vi "Read AI and Write AO.vi"(8 "error in (no error)":errorcluster, 10 "AO []":waveform(dbl)[](array[waveform]), 11 "LockinDAQ":refnum<class "LockinDAQ.lvclass">) -> (0 "error out":errorcluster, 2 "AI []":waveform(dbl)[](array[waveform]), 3 "LockinDAQ out":refnum<class "LockinDAQ.lvclass">)   [LabVIEW 2016, in "LockinDAQ.lvclass"]
uses:
  LockinDAQ.lvclass
  LockinDAQ.lvclass/LockinDAQ.ctl
  Typedefs/DAQType-enum.ctl
  <vilib>/DAQmx/write.llb/DAQmx Write (Analog 1D Wfm NChan NSamp).vi
  <vilib>/DAQmx/read.llb/DAQmx Read (Analog 1D Wfm NChan NSamp).vi
  <vilib>/DAQmx/miscellaneous.llb/DAQmx Fill In Error Info.vi
  <resource>/objmgr/daqmx.rc
panel:
  out "Numeric":i32
  out "AvailSampPerChan 4":u32
  out "AvailSampPerChan 3":u32
  out "AvailSampPerChan 2":u32
  out "AvailSampPerChan 1":u32
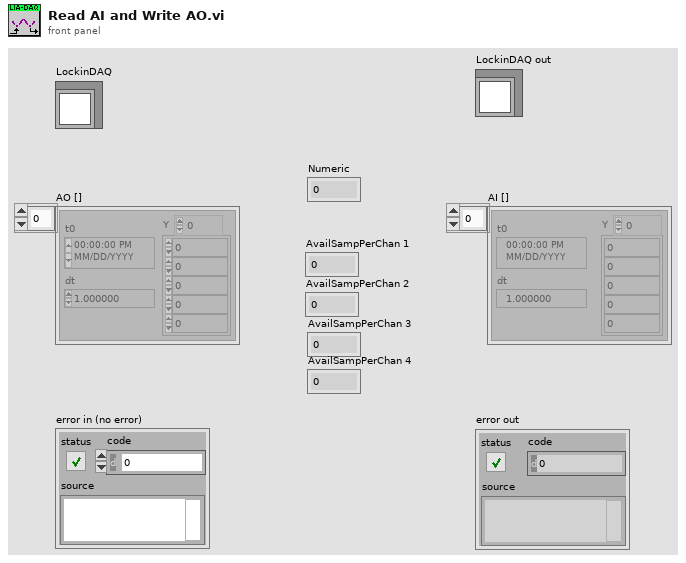
[diagram p1: front panel]
types:
  T1 = typedef "LockinDAQ.lvclass/DAQType-enum.ctl" = enum16{"None", "USB 4431", "PXI 446x"}
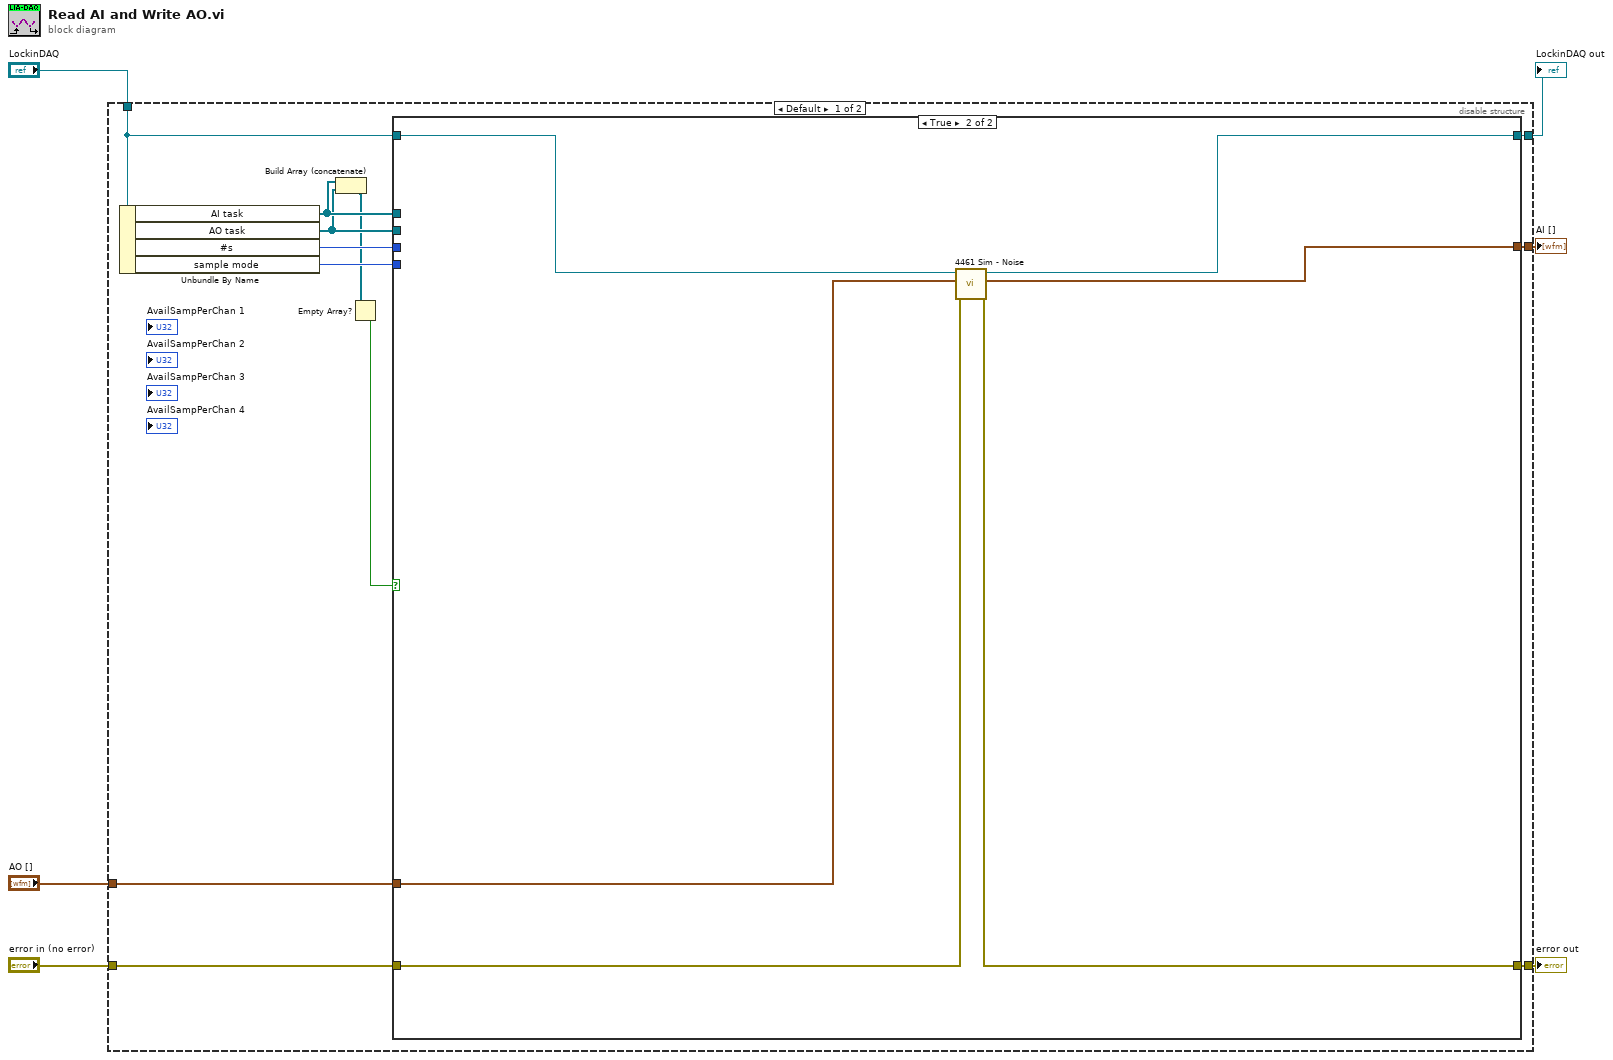
[diagram p0: block diagram]
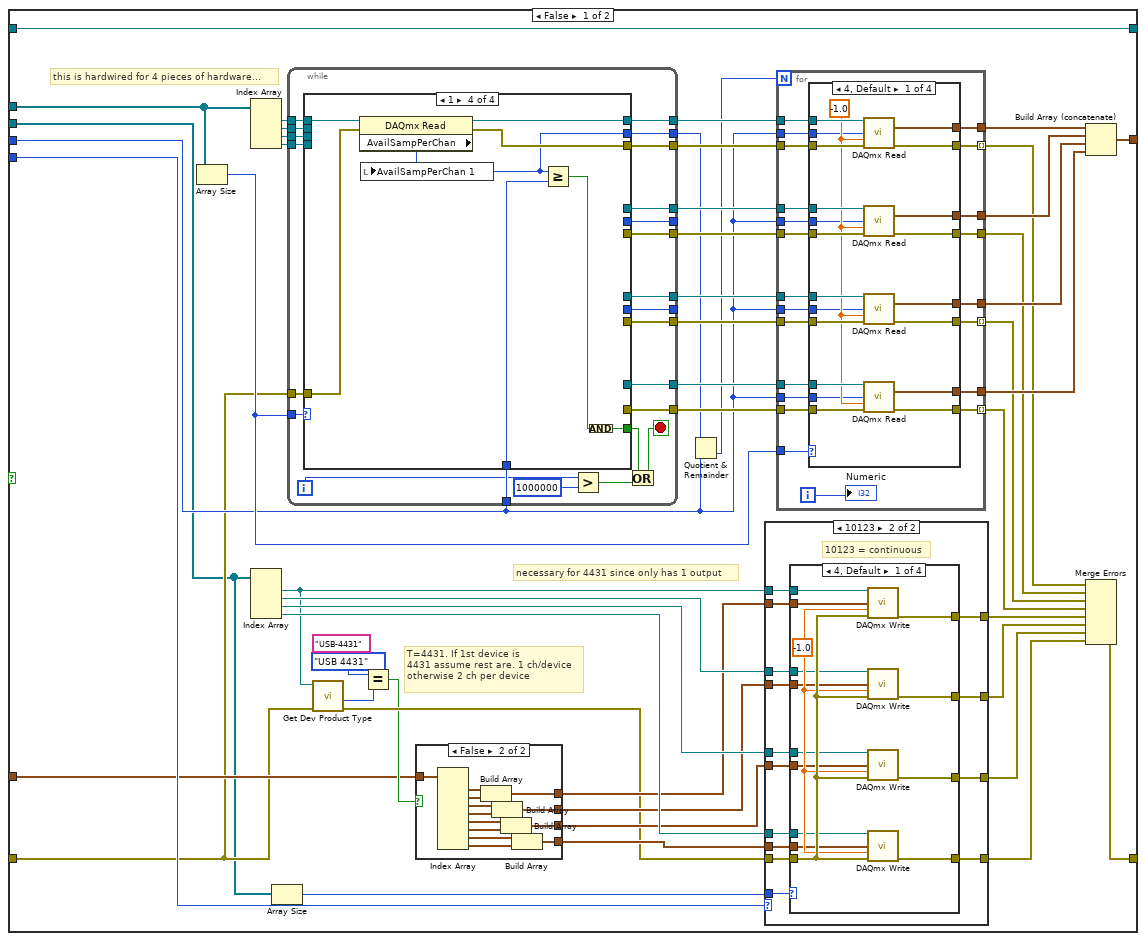
[diagram p2: hidden frame]
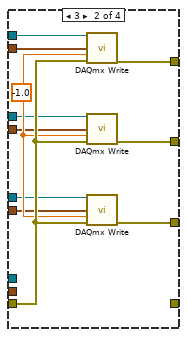
[diagram p4: hidden frame]
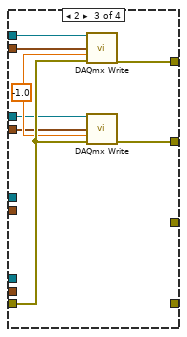
[diagram p5: hidden frame]
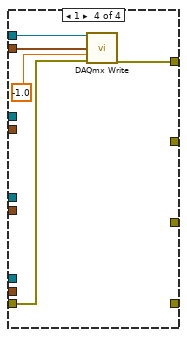
[diagram p6: hidden frame]
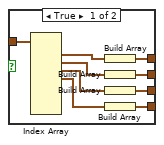
[diagram p7: hidden frame]
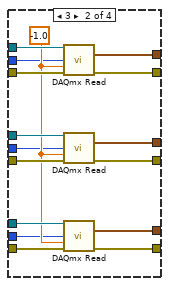
[diagram p8: hidden frame]
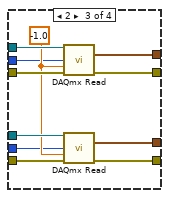
[diagram p9: hidden frame]
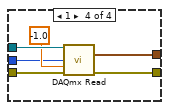
[diagram p10: hidden frame]
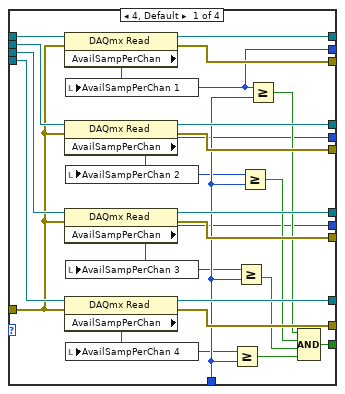
[diagram p11: hidden frame]
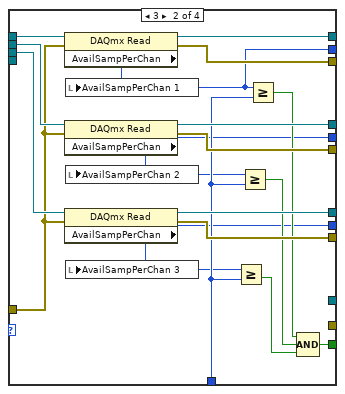
[diagram p12: hidden frame]
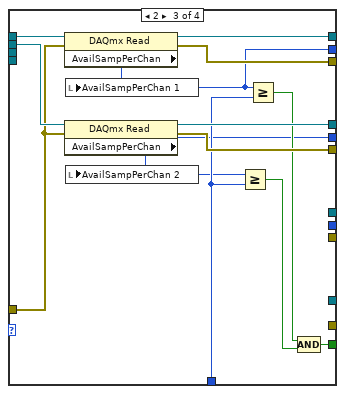
[diagram p13: hidden frame]
diagram:
  n1 = disable-structure shown="Default" {
    disable-tunnel: [w18 w309] -> w6
    disable-tunnel: [w15 w310] -> w5
    disable-tunnel: "LockinDAQ" -> [w8 _]
    disable-tunnel: "AO []" -> [w14 w309]
    disable-tunnel: "error in (no error)" -> [w13 w310]
    disable-tunnel: [w7 _] -> w1
    frame condition #0 (active) {
      n2 = Unbundle By Name(w8) -> ("AI task"=w12:refnum<k21>[], "AO task"=w11:refnum<k21>[], "#s"=w17:i32, "sample mode"=w16:i32)
      n3 = Build Array (concatenate)(w12, w11) -> (w10:refnum<k21>[])
      n4 = Empty Array?(array=w10) -> (empty?=w9:bool)
      n5 = case shown="True" w9 {
        tunnel: [w67 w306] -> w18
        tunnel: w17 -> [w29 _]
        tunnel: w16 -> [w28 _]
        tunnel: [w27 w304] -> w15
        tunnel: w14 -> [w26 w303]
        tunnel: w13 -> [w25 w305]
        tunnel: w12 -> [w21 _]
        tunnel: w11 -> [w20 _]
        tunnel: w8 -> [w19 w308]
        tunnel: [w19 w307] -> w7
        frame False {
          (unwired) "USB-4431" ("ProductType")
          # "this is hardwired for 4 pieces of hardware..."
          # "T=4431. If 1st device is \n4431 assume rest are. 1 ch/device\notherwise 2 ch per device"
          # "necessary for 4431 since only has 1 output"
          n6 = Array Size(array=w21) -> (size(s)=w35:i32)
          n7 = Index Array(array=w21) -> (element #1=w63:refnum<k21>, element #2=w64:refnum<k21>, element #3=w65:refnum<k21>, element #4=w66:refnum<k21>)  [unwired: 4 in]
          n8 = Index Array(array=w20) -> (element #1=w43:refnum<k21>, element #2=w54:refnum<k21>, element #3=w53:refnum<k21>, element #4=w52:refnum<k21>)  [unwired: 4 in]
          n9 = Array Size(array=w20) -> (size(s)=w44:i32)
          n10 = while {
            tunnel: w66 -> [w240]
            tunnel: w65 -> [w239]
            tunnel: w64 -> [w238]
            tunnel: w63 -> [w237]
            tunnel: [w236] -> w62
            tunnel: [w235] -> w61
            tunnel: [w234] -> w60
            tunnel: [w233] -> w59
            tunnel: w25 -> [w228]
            tunnel: [w232] -> w58
            tunnel: [w231] -> w57
            tunnel: [w230] -> w56
            tunnel: [w229] -> w55
            tunnel: w29 -> [w227]
            tunnel: [w224] -> w45
            tunnel: [w226] -> _
            tunnel: [w225] -> _
            tunnel: w35 -> [w223]
            i -> [w220]
            stop <- w221 stop-if-true
            n11 = case shown="1" w223 {
              tunnel: w240 -> [w263 _ _ _]
              tunnel: w239 -> [w262 w281 _ _]
              tunnel: w238 -> [w261 w280 w294 _]
              tunnel: w237 -> [w260 w279 w293 w302]
              tunnel: [w259 w278 w292 w301] -> w236
              tunnel: [w258 w277 w291 _] -> w235
              tunnel: [w257 w276 _ _] -> w234
              tunnel: [w256 _ _ _] -> w233
              tunnel: [w255 w275 w290 w300] -> w232
              tunnel: [w254 w274 w289 _] -> w231
              tunnel: [w253 w273 _ _] -> w230
              tunnel: [w252 _ _ _] -> w229
              tunnel: w228 -> [w251 w272 w288 w299]
              tunnel: w227 -> [w246 w268 w285 w297]
              tunnel: [w241 w264 w282 w295] -> w222
              tunnel: [w244 w267 _ _] -> w226
              tunnel: [w243 w266 w284 _] -> w225
              tunnel: [w242 w265 w283 w296] -> w224
              frame 4, Default {
                n12 = property class="DAQmx Read"(reference=w260, error in=w251) -> (reference out=w259:refnum<k21>, error out=w255:errorcluster, "AvailSampPerChan"=w242:u32)
                n13 = property class="DAQmx Read"(reference=w261, error in=w251) -> (reference out=w258:refnum<k21>, error out=w254:errorcluster, "AvailSampPerChan"=w243:u32)
                n14 = property class="DAQmx Read"(reference=w262, error in=w251) -> (reference out=w257:refnum<k21>, error out=w253:errorcluster, "AvailSampPerChan"=w244:u32)
                n15 = property class="DAQmx Read"(reference=w263, error in=w251) -> (reference out=w256:refnum<k21>, error out=w252:errorcluster, "AvailSampPerChan"=w245:u32)
                n16 = local write "AvailSampPerChan 1"(w242) -> ()
                n17 = local write "AvailSampPerChan 2"(w243) -> ()
                n18 = local write "AvailSampPerChan 3"(w244) -> ()
                n19 = local write "AvailSampPerChan 4"(w245) -> ()
                n20 = Greater Or Equal?(x=w245, y=w246) -> (x >= y?=w250:bool)
                n21 = Greater Or Equal?(x=w244, y=w246) -> (x >= y?=w249:bool)
                n22 = Greater Or Equal?(x=w243, y=w246) -> (x >= y?=w248:bool)
                n23 = Greater Or Equal?(x=w242, y=w246) -> (x >= y?=w247:bool)
                n24 = Compound Arithmetic op=AND(w247, w248, w249, w250) -> (w241:bool)
              }
              frame 3 {
                n25 = property class="DAQmx Read"(reference=w279, error in=w272) -> (reference out=w278:refnum<k21>, error out=w275:errorcluster, "AvailSampPerChan"=w265:u32)
                n26 = property class="DAQmx Read"(reference=w280, error in=w272) -> (reference out=w277:refnum<k21>, error out=w274:errorcluster, "AvailSampPerChan"=w266:u32)
                n27 = property class="DAQmx Read"(reference=w281, error in=w272) -> (reference out=w276:refnum<k21>, error out=w273:errorcluster, "AvailSampPerChan"=w267:u32)
                n28 = local write "AvailSampPerChan 1"(w265) -> ()
                n29 = local write "AvailSampPerChan 2"(w266) -> ()
                n30 = local write "AvailSampPerChan 3"(w267) -> ()
                n31 = Greater Or Equal?(x=w267, y=w268) -> (x >= y?=w271:bool)
                n32 = Greater Or Equal?(x=w266, y=w268) -> (x >= y?=w270:bool)
                n33 = Greater Or Equal?(x=w265, y=w268) -> (x >= y?=w269:bool)
                n34 = Compound Arithmetic op=AND(w269, w270, w271) -> (w264:bool)
              }
              frame 2 {
                n35 = property class="DAQmx Read"(reference=w293, error in=w288) -> (reference out=w292:refnum<k21>, error out=w290:errorcluster, "AvailSampPerChan"=w283:u32)
                n36 = property class="DAQmx Read"(reference=w294, error in=w288) -> (reference out=w291:refnum<k21>, error out=w289:errorcluster, "AvailSampPerChan"=w284:u32)
                n37 = local write "AvailSampPerChan 1"(w283) -> ()
                n38 = local write "AvailSampPerChan 2"(w284) -> ()
                n39 = Greater Or Equal?(x=w284, y=w285) -> (x >= y?=w287:bool)
                n40 = Greater Or Equal?(x=w283, y=w285) -> (x >= y?=w286:bool)
                n41 = Compound Arithmetic op=AND(w286, w287) -> (w282:bool)
              }
              frame 1 {
                n42 = property class="DAQmx Read"(reference=w302, error in=w299) -> (reference out=w301:refnum<k21>, error out=w300:errorcluster, "AvailSampPerChan"=w296:u32)
                n43 = local write "AvailSampPerChan 1"(w296) -> ()
                n44 = Greater Or Equal?(x=w296, y=w297) -> (x >= y?=w298:bool)
                n45 = Compound Arithmetic op=AND(w298) -> (w295:bool)
              }
            }
            n46 = Greater?(x=w220, y=1000000) -> (0:w218:bool)
            n47 = Or(x=w222, y=w218) -> (x .or. y?=w221:bool)
          }
          n48 = call "Get Dev Product Type.vi"("error in (no error)"=w25, "Refnum in"=w43) -> ("error out"=w37:errorcluster, "DAQ Type"=w38:T1)  [unwired: 6 in, 2 out]
          n49 = Equal?(x=DAQType-enum."USB 4431", y=w38) -> (x = y?=w36:bool)
          n50 = case shown="False" w36 {
            tunnel: [w128 w134] -> w40
            tunnel: [w127 w133] -> w41
            tunnel: [w126 w132] -> w42
            tunnel: [w124 w130] -> w39
            tunnel: w26 -> [w123 w129]
            frame True {
              n51 = Index Array(array=w123) -> (element #1=w125:waveform(dbl), element #2=w122:waveform(dbl), element #3=w121:waveform(dbl), element #4=w120:waveform(dbl))  [unwired: 8 in, 4 out]
              n52 = Build Array(w125) -> (w124:waveform(dbl)[])
              n53 = Build Array(w122) -> (w128:waveform(dbl)[])
              n54 = Build Array(w121) -> (w127:waveform(dbl)[])
              n55 = Build Array(w120) -> (w126:waveform(dbl)[])
            }
            frame False {
              n56 = Index Array(array=w129) -> (element #1=w131:waveform(dbl), element #2=w141:waveform(dbl), element #3=w140:waveform(dbl), element #4=w139:waveform(dbl), element #5=w138:waveform(dbl), element #6=w137:waveform(dbl), element #7=w136:waveform(dbl), element #8=w135:waveform(dbl))  [unwired: 8 in]
              n57 = Build Array(w131, w141) -> (w130:waveform(dbl)[])
              n58 = Build Array(w140, w139) -> (w134:waveform(dbl)[])
              n59 = Build Array(w138, w137) -> (w133:waveform(dbl)[])
              n60 = Build Array(w136, w135) -> (w132:waveform(dbl)[])
            }
          }
          n61 = Quotient & Remainder(x=w45, y=w29) -> (floor(x/y)=w46:u32)  [unwired: 1 out]
          n62 = case shown="10123" w28 {
            tunnel: w54 -> [_ w81]
            tunnel: w53 -> [_ w80]
            tunnel: w52 -> [_ w79]
            tunnel: [_ w78] -> w51
            tunnel: [_ w77] -> w24
            tunnel: [_ w76] -> w23
            tunnel: [_ w75] -> w22
            tunnel: w44 -> [_ w74]
            tunnel: w43 -> [_ w73]
            tunnel: w42 -> [_ w72]
            tunnel: w41 -> [_ w71]
            tunnel: w40 -> [_ w70]
            tunnel: w39 -> [_ w69]
            tunnel: w37 -> [_ w68]
            frame 10178, Default {
              # "10178 = finite sample mode (IV\nmode). Do not try to write\nmore samples to the buffer"
            }
            frame 10123 {
              # "10123 = continuous"
              n63 = case shown="4, Default" w74 {
                tunnel: w68 -> [w95 w106 w114 w119]
                tunnel: w81 -> [w93 w104 w112 _]
                tunnel: w80 -> [w92 w103 _ _]
                tunnel: w79 -> [w91 _ _ _]
                tunnel: w70 -> [w90 w102 w111 _]
                tunnel: w71 -> [w89 w101 _ _]
                tunnel: w72 -> [w88 _ _ _]
                tunnel: [w87 w100 w110 w117] -> w78
                tunnel: [w86 w99 w109 _] -> w77
                tunnel: [w85 w98 _ _] -> w76
                tunnel: [w84 _ _ _] -> w75
                tunnel: w73 -> [w83 w97 w108 w116]
                tunnel: w69 -> [w82 w96 w107 w115]
                frame 4, Default {
                  w94 = -1.0 ("timeout")
                  n64 = call-poly <vilib>:"DAQmx Write.vi"("task/channels in"=w83, "data"=w82, "timeout"=w94, "error in"=w95) -> ("error out"=w87:errorcluster)  [unwired: 9 in, 2 out]
                  n65 = call-poly <vilib>:"DAQmx Write.vi"("task/channels in"=w93, "data"=w90, "timeout"=w94, "error in"=w95) -> ("error out"=w86:errorcluster)  [unwired: 9 in, 2 out]
                  n66 = call-poly <vilib>:"DAQmx Write.vi"("task/channels in"=w92, "data"=w89, "timeout"=w94, "error in"=w95) -> ("error out"=w85:errorcluster)  [unwired: 9 in, 2 out]
                  n67 = call-poly <vilib>:"DAQmx Write.vi"("task/channels in"=w91, "data"=w88, "timeout"=w94, "error in"=w95) -> ("error out"=w84:errorcluster)  [unwired: 9 in, 2 out]
                }
                frame 3 {
                  w105 = -1.0 ("timeout")
                  n68 = call-poly <vilib>:"DAQmx Write.vi"("task/channels in"=w97, "data"=w96, "timeout"=w105, "error in"=w106) -> ("error out"=w100:errorcluster)  [unwired: 9 in, 2 out]
                  n69 = call-poly <vilib>:"DAQmx Write.vi"("task/channels in"=w104, "data"=w102, "timeout"=w105, "error in"=w106) -> ("error out"=w99:errorcluster)  [unwired: 9 in, 2 out]
                  n70 = call-poly <vilib>:"DAQmx Write.vi"("task/channels in"=w103, "data"=w101, "timeout"=w105, "error in"=w106) -> ("error out"=w98:errorcluster)  [unwired: 9 in, 2 out]
                }
                frame 2 {
                  w113 = -1.0 ("timeout")
                  n71 = call-poly <vilib>:"DAQmx Write.vi"("task/channels in"=w108, "data"=w107, "timeout"=w113, "error in"=w114) -> ("error out"=w110:errorcluster)  [unwired: 9 in, 2 out]
                  n72 = call-poly <vilib>:"DAQmx Write.vi"("task/channels in"=w112, "data"=w111, "timeout"=w113, "error in"=w114) -> ("error out"=w109:errorcluster)  [unwired: 9 in, 2 out]
                }
                frame 1 {
                  n73 = call-poly <vilib>:"DAQmx Write.vi"("task/channels in"=w116, "data"=w115, "timeout"=-1.0, "error in"=w119) -> ("error out"=w117:errorcluster)  [unwired: 9 in, 2 out]
                }
              }
            }
          }
          n74 = for {
            N: w46 -> [_]
            tunnel: w62 -> [w163]
            tunnel: w61 -> [w162]
            tunnel: w60 -> [w161]
            tunnel: w59 -> [w160]
            tunnel: w58 -> [w159]
            tunnel: w57 -> [w158]
            tunnel: w56 -> [w157]
            tunnel: w55 -> [w156]
            tunnel: [w155] -> w50
            tunnel: [w154] -> w49
            tunnel: [w153] -> w48
            tunnel: [w152] -> w47
            tunnel: w29 -> [w151]
            tunnel: w29 -> [w150]
            tunnel: w29 -> [w149]
            tunnel: w29 -> [w148]
            tunnel: [w147] -> w32 mode=indexing
            tunnel: [w146] -> w33
            tunnel: [w145] -> w34 mode=indexing
            tunnel: [w144] -> w31 mode=indexing
            tunnel: w35 -> [w142]
            i -> [w143]
            n75 = case shown="4, Default" w142 {
              tunnel: w163 -> [w184 w200 w211 w217]
              tunnel: w162 -> [w183 w199 w210 _]
              tunnel: w161 -> [w182 w198 _ _]
              tunnel: w160 -> [w181 _ _ _]
              tunnel: w159 -> [w180 w197 w209 w216]
              tunnel: w158 -> [w179 w196 w208 _]
              tunnel: w157 -> [w178 w195 _ _]
              tunnel: w156 -> [w177 _ _ _]
              tunnel: [w175 w193 w206 _] -> w155
              tunnel: [w174 w192 w205 w214] -> w154
              tunnel: [w173 w191 _ _] -> w153
              tunnel: [w172 _ _ _] -> w152
              tunnel: w151 -> [w171 _ _ _]
              tunnel: w150 -> [w170 w190 w204 w213]
              tunnel: w149 -> [w169 w189 _ _]
              tunnel: w148 -> [w168 w188 w203 _]
              tunnel: [w167 w187 w202 w212] -> w147
              tunnel: [w166 w186 w201 _] -> w146
              tunnel: [w165 w185 _ _] -> w145
              tunnel: [w164 _ _ _] -> w144
              frame 4, Default {
                w176 = -1.0 ("timeout")
                n76 = call-poly <vilib>:"DAQmx Read.vi"("task/channels in"=w184, "number of samples per channel"=w170, "timeout"=w176, "error in"=w180) -> ("data"=w174:waveform(dbl)[], "error out"=w167:errorcluster)  [unwired: 9 in, 1 out]
                n77 = call-poly <vilib>:"DAQmx Read.vi"("task/channels in"=w183, "number of samples per channel"=w168, "timeout"=w176, "error in"=w179) -> ("data"=w175:waveform(dbl)[], "error out"=w166:errorcluster)  [unwired: 9 in, 1 out]
                n78 = call-poly <vilib>:"DAQmx Read.vi"("task/channels in"=w182, "number of samples per channel"=w169, "timeout"=w176, "error in"=w178) -> ("data"=w173:waveform(dbl)[], "error out"=w165:errorcluster)  [unwired: 9 in, 1 out]
                n79 = call-poly <vilib>:"DAQmx Read.vi"("task/channels in"=w181, "number of samples per channel"=w171, "timeout"=w176, "error in"=w177) -> ("data"=w172:waveform(dbl)[], "error out"=w164:errorcluster)  [unwired: 9 in, 1 out]
              }
              frame 3 {
                w194 = -1.0 ("timeout")
                n80 = call-poly <vilib>:"DAQmx Read.vi"("task/channels in"=w200, "number of samples per channel"=w190, "timeout"=w194, "error in"=w197) -> ("data"=w192:waveform(dbl)[], "error out"=w187:errorcluster)  [unwired: 9 in, 1 out]
                n81 = call-poly <vilib>:"DAQmx Read.vi"("task/channels in"=w199, "number of samples per channel"=w188, "timeout"=w194, "error in"=w196) -> ("data"=w193:waveform(dbl)[], "error out"=w186:errorcluster)  [unwired: 9 in, 1 out]
                n82 = call-poly <vilib>:"DAQmx Read.vi"("task/channels in"=w198, "number of samples per channel"=w189, "timeout"=w194, "error in"=w195) -> ("data"=w191:waveform(dbl)[], "error out"=w185:errorcluster)  [unwired: 9 in, 1 out]
              }
              frame 2 {
                w207 = -1.0 ("timeout")
                n83 = call-poly <vilib>:"DAQmx Read.vi"("task/channels in"=w211, "number of samples per channel"=w204, "timeout"=w207, "error in"=w209) -> ("data"=w205:waveform(dbl)[], "error out"=w202:errorcluster)  [unwired: 9 in, 1 out]
                n84 = call-poly <vilib>:"DAQmx Read.vi"("task/channels in"=w210, "number of samples per channel"=w203, "timeout"=w207, "error in"=w208) -> ("data"=w206:waveform(dbl)[], "error out"=w201:errorcluster)  [unwired: 9 in, 1 out]
              }
              frame 1 {
                n85 = call-poly <vilib>:"DAQmx Read.vi"("task/channels in"=w217, "number of samples per channel"=w213, "timeout"=-1.0, "error in"=w216) -> ("data"=w214:waveform(dbl)[], "error out"=w212:errorcluster)  [unwired: 9 in, 1 out]
              }
            }
            "Numeric" <- w143
          }
          n86 = Build Array (concatenate)(w49, w50, w48, w47) -> (w67:waveform(dbl)[])
          n87 = Merge Errors(w32, w33, w34, w31, w51, w24, w23, w22) -> (w27:errorcluster)
        }
        frame True {
          n88 = call "4461 Sim - Noise.vi"("error in (no error)"=w305, "AO []"=w303, "LockinDAQ"=w308) -> ("error out"=w304:errorcluster, "\"AI\" []"=w306:waveform(dbl)[], "LockinDAQ out"=w307:refnum<class "LockinDAQ.lvclass">)  [unwired: 6 in]
        }
      }
    }
    frame condition #1 {
    }
  }
  "AI []" <- w6
  "error out" <- w5
  "LockinDAQ out" <- w1
